vi "Init Visa.vi"(8 "error in (no error)":errorcluster, 10 "Baud (115200)":u32=115200, 11 "VISA resource name in":refnum<visa-resource-name>) -> (0 "error out":errorcluster, 3 "VisaSession out":refnum<class "VisaSession.lvclass">)   [LabVIEW 2020, in "CTI.lvlib" / "VisaSession.lvclass"]
uses:
  VisaSession.lvclass
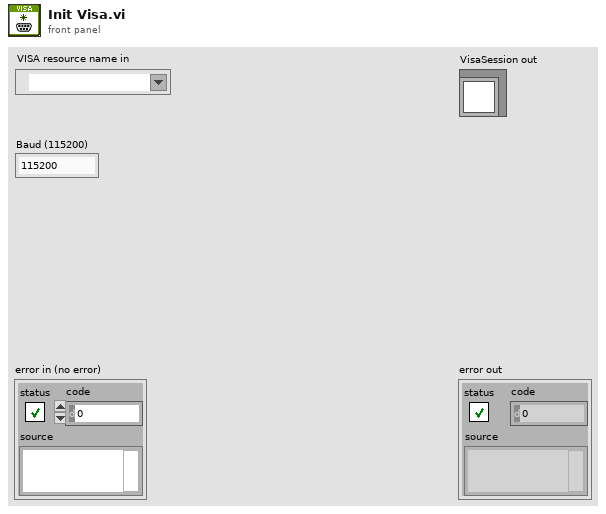
[diagram p1: front panel]
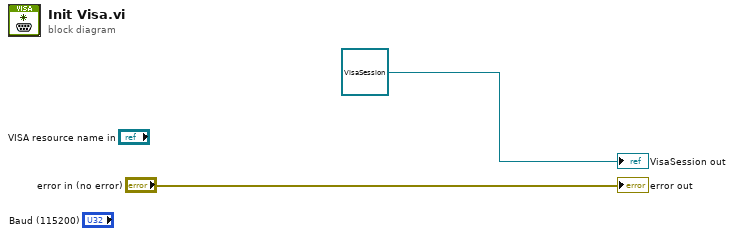
[diagram p0: block diagram]
diagram:
  "error out" <- "error in (no error)"
  "VisaSession out" <- refnum<class "VisaSession.lvclass"> refnum ("VisaSession in")
